vi "Loop_Auto.vi"() -> ()   [LabVIEW 2017, in "Autonomous.lvlib"]
uses:
  Autonomous.lvlib
  ENUM_Auto_State.ctl
  TypeDef/CLUSTER_CMD_WC_Drive.ctl
  TypeDef/ENUM_WC_Drive_DriveMode.ctl
  TypeDef/CLUSTER_Drive_ACT Loop_VBus Data.ctl
  TypeDef/CLUSTER_X and Y.ctl
  TypeDef/CLUSTER_Drive_ACT Loop_Profile Data.ctl
  ENUM_Auto_Action.ctl
  _SHARE ALL/Global Share All/Global_STOP.vi
  Globals/Global_CMD_Drive.vi
panel:
  out "Cycle Time (S)":dbl format="%.3g"
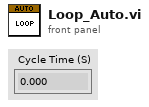
[diagram p1: front panel]
types:
  T1 = typedef "CLUSTER_CMD_WC_Drive.ctl" = cluster{"Drive_Mode":T2, "VBus":T3, "Profile":T5, "Zero Drive Encoders":bool, "Set Target Position(IN)":dbl, "Target Angle(Degree)":dbl, "Lock Angle":bool, "Zero YAW":bool}
  T2 = typedef "ENUM_WC_Drive_DriveMode.ctl" = enum16{"Motion Profile", "CrossLineAuto", "VBus", "Stop"}
  T3 = typedef "CLUSTER_Drive_ACT Loop_VBus Data.ctl" = cluster{"Drive":T4, "Turbo":bool}
  T4 = typedef "CLUSTER_X and Y.ctl" = cluster{"Steer":dbl, "Throtle":dbl}
  T5 = typedef "CLUSTER_Drive_ACT Loop_Profile Data.ctl" = cluster{"Start":bool}
  T6 = typedef "Autonomous.lvlib/ENUM_Auto_State.ctl" = enum16{"Startup", "Idle", "Cross Line", "Shutdown"}
  T7 = typedef "Autonomous.lvlib/ENUM_Auto_Action.ctl" = enum16{"No Action", "Reset Time", "Reset All", "Lock Angle", "Drive", "Zero Drive Encoders", "Zero YAW"}
  T8 = cluster{"State":T6, "Previous State":T6, "Current Time":timestamp, "Previous Time":timestamp, "Start Time":timestamp, "Target Time (ms)":u32, "Cycle Time(S)":dbl, "CMD_Drive_Data":T1, "Test":dbl, "Steering":dbl, "Throtal":dbl, "Encoder Target Position(in)":dbl, "Zero Drive Encoders":bool, "Lock Angle":bool, "Target Angle(Degree)":dbl, "Zero YAW":bool}
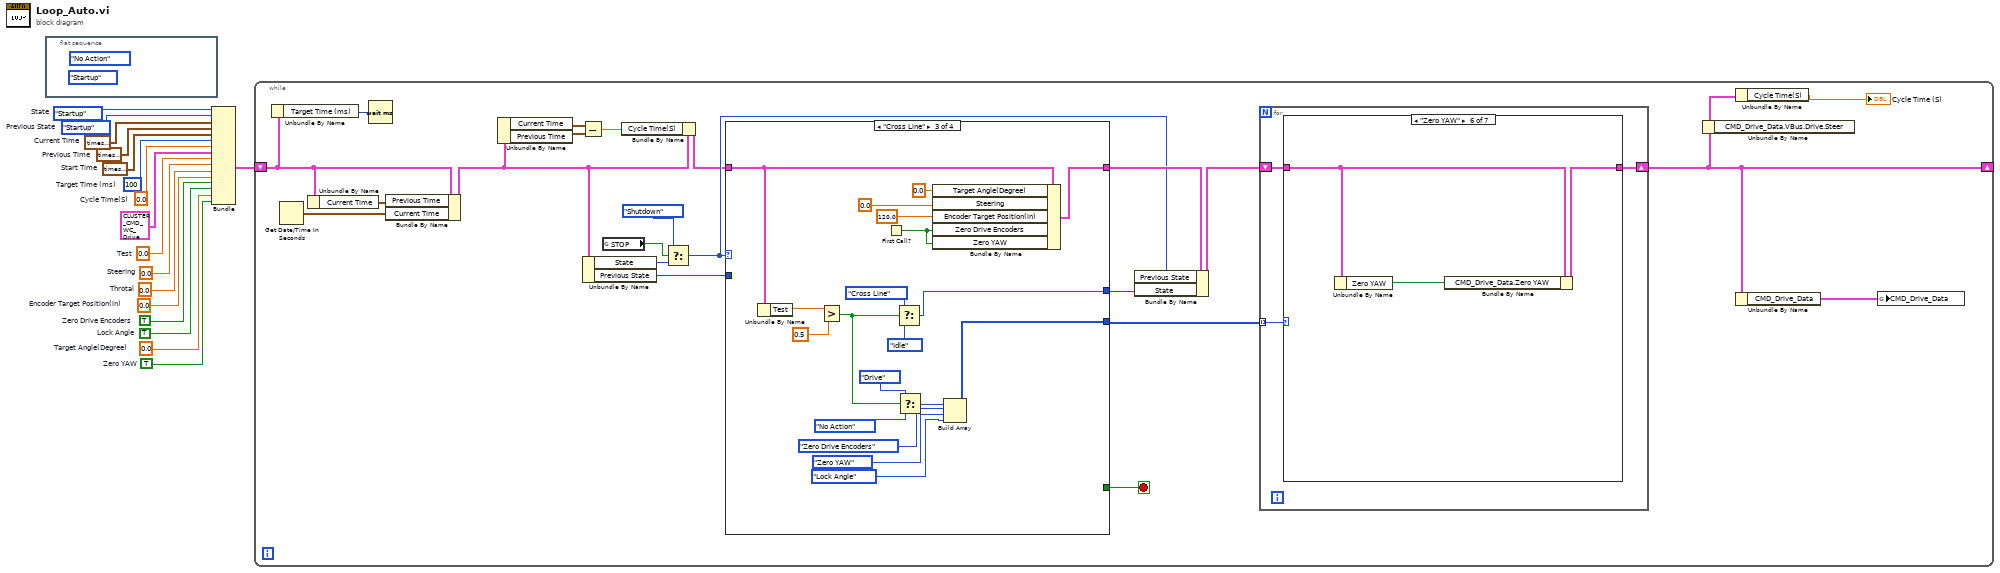
[diagram p0: block diagram]
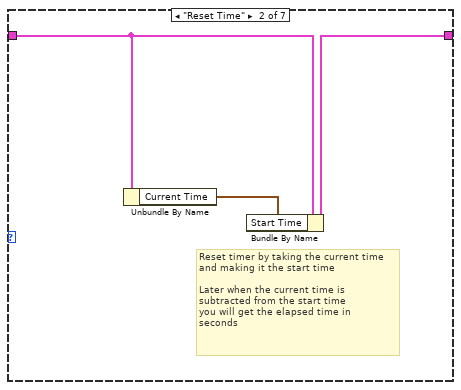
[diagram p3: hidden frame]
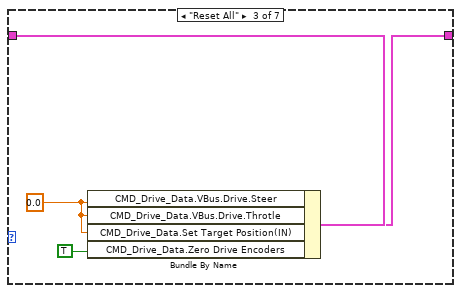
[diagram p4: hidden frame]
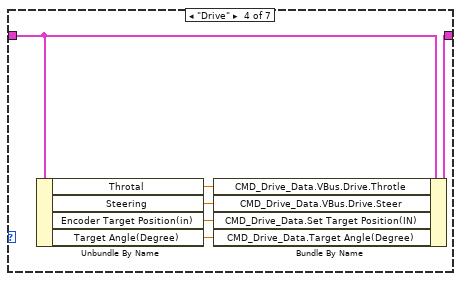
[diagram p5: hidden frame]
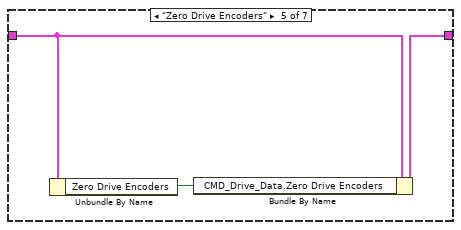
[diagram p6: hidden frame]
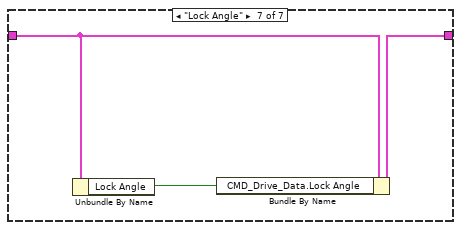
[diagram p7: hidden frame]
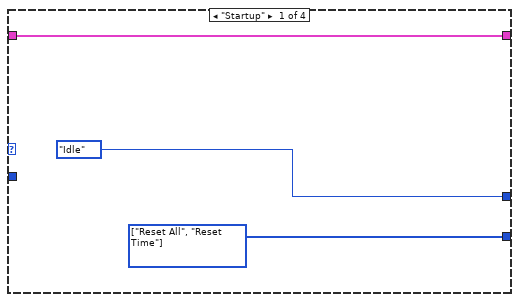
[diagram p8: hidden frame]
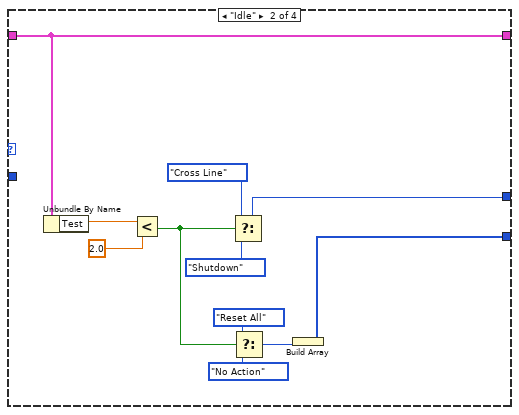
[diagram p9: hidden frame]
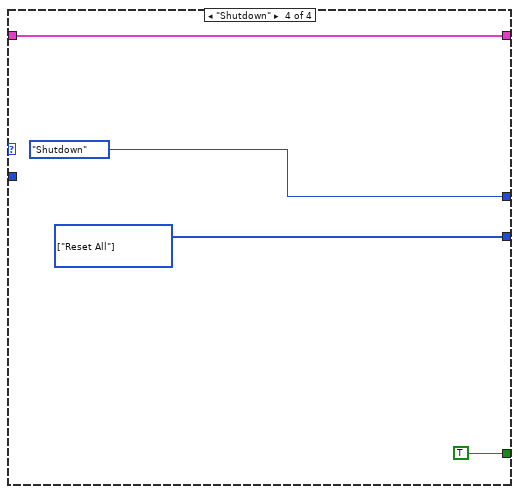
[diagram p10: hidden frame]
diagram:
  w1 = TRUE  # Zero YAW
  w2 = 0.0  # Target Angle(Degree)
  w3 = TRUE  # Lock Angle
  w4 = TRUE  # Zero Drive Encoders
  w5 = 0.0  # Encoder Target Position(in)
  w6 = 0.0  # Throtal
  w7 = 0.0  # Steering
  w8 = 0.0  # Test
  w10 = 0.0  # Cycle Time(S)
  w11 = ENUM_Auto_State."Startup"  # Previous State
  w12 = timestamp(0 s since 1904-01-01)  # Previous Time
  w13 = u32 100  # Target Time (ms)
  w14 = timestamp(0 s since 1904-01-01)  # Start Time
  w15 = timestamp(0 s since 1904-01-01)  # Current Time
  w16 = ENUM_Auto_State."Startup"  # State
  n1 = flat-sequence {
    frame #0 {
      (unwired) ENUM_Auto_State."Startup" ("State")
      (unwired) ENUM_Auto_Action."No Action" ("Action")
    }
  }
  n2 = Bundle("State"=w16, "Previous State"=w11, "Current Time"=w15, "Previous Time"=w12, "Start Time"=w14, "Target Time (ms)"=w13, "Cycle Time(S)"=w10, "CMD_Drive_Data"=T1 {"Drive_Mode"=enum."Motion Profile", "VBus"={"Drive"={"Steer"=0.0, "Throtle"=0.0}, "Turbo"=FALSE}, "Profile"={"Start"=FALSE}, "Zero Drive Encoders"=FALSE, "Set Target Position(IN)"=0.0, "Target Angle(Degree)"=0.0, "Lock Angle"=FALSE, "Zero YAW"=FALSE}, "Test"=w8, "Steering"=w7, "Throtal"=w6, "Encoder Target Position(in)"=w5, "Zero Drive Encoders"=w4, "Lock Angle"=w3, "Target Angle(Degree)"=w2, "Zero YAW"=w1) -> (w17:T8)  [unwired: 1 in]
  n3 = while {
    shift-right: [w27] -> _
    shift-left: w17 -> [w30]
    stop <- w19 stop-if-true
    n4 = Unbundle By Name(w30) -> ("Target Time (ms)"=w32:u32)
    n5 = Get Date/Time In Seconds() -> (seconds since 1Jan1904=w39:timestamp)
    n6 = Unbundle By Name(w30) -> ("Current Time"=w31:timestamp)
    n7 = Wait (ms)(milliseconds to wait=w32) -> ()  [unwired: 1 out]
    n8 = Bundle By Name(cluster=w30, "Previous Time"=w31, "Current Time"=w39) -> (w23:T8)
    n9 = Unbundle By Name(w23) -> ("Current Time"=w24:timestamp, "Previous Time"=w25:timestamp)
    n10 = Subtract(x=w24, y=w25) -> (x-y=w21:dbl)
    n11 = Unbundle By Name(w23) -> ("State"=w33:T6, "Previous State"=w29:T6)
    n12 = global read "Global_STOP.vi" "STOP"() -> (w35:bool)
    n13 = Bundle By Name(cluster=w23, "Cycle Time(S)"=w21) -> (w22:T8)
    n14 = Select(t=ENUM_Auto_State."Shutdown" ("State"), s=w35, f=w33) -> (s? t:f=w28:T6)
    n15 = case shown="\"Cross Line\"" w28 {
      tunnel: w22 -> [w68 w79 w88 w102]
      tunnel: [w68 w79 w87 w102] -> w37
      tunnel: [ENUM_Auto_State."Idle" ("State") w78 w98 ENUM_Auto_State."Shutdown" ("State")] -> w36
      tunnel: [w67 w71 w91 w100] -> w20
      tunnel: w29 -> [_ _ _ _]
      tunnel: [_ _ _ TRUE] -> w19
      frame "Startup" {
        w67 = T7[] [enum."Reset All", enum."Reset Time"] items=["No Action", "Reset Time", "Reset All", "Lock Angle", "Drive", "Zero Drive Encoders", "Zero YAW"] ("Actions")
      }
      frame "Idle" {
        n16 = Unbundle By Name(w79) -> ("Test"=w70:dbl)
        n17 = Less?(x=w70, y=2.0) -> (x < y?=w73:bool)
        n18 = Select(t=ENUM_Auto_State."Cross Line" ("State"), s=w73, f=ENUM_Auto_State."Shutdown" ("State")) -> (s? t:f=w78:T6)
        n19 = Select(t=ENUM_Auto_Action."Reset All" ("Action"), s=w73, f=ENUM_Auto_Action."No Action" ("Action")) -> (s? t:f=w72:T7)
        n20 = Build Array(w72) -> (w71:T7[])
      }
      frame "Cross Line" {
        n21 = Unbundle By Name(w88) -> ("Test"=w90:dbl)
        n22 = Greater?(x=w90, y=0.5) -> (0:w93:bool)
        n23 = First Call?() -> (First Call?: T/F=w82:bool)
        n24 = Select(t=ENUM_Auto_State."Cross Line" ("State"), s=w93, f=ENUM_Auto_State."Idle" ("State")) -> (s? t:f=w98:T6)
        n25 = Select(t=ENUM_Auto_Action."Drive" ("Action"), s=w93, f=ENUM_Auto_Action."No Action" ("Action")) -> (s? t:f=w92:T7)
        n26 = Bundle By Name(cluster=w88, "Target Angle(Degree)"=0.0, "Steering"=0.0, "Encoder Target Position(in)"=120.0, "Zero Drive Encoders"=w82, "Zero YAW"=w82) -> (w87:T8)
        n27 = Build Array(w92, ENUM_Auto_Action."Zero Drive Encoders" ("Action"), ENUM_Auto_Action."Zero YAW" ("Action"), ENUM_Auto_Action."Lock Angle" ("Action")) -> (w91:T7[])
      }
      frame "Shutdown" {
        w100 = T7[] [enum."Reset All"] items=["No Action", "Reset Time", "Reset All", "Lock Angle", "Drive", "Zero Drive Encoders", "Zero YAW"] ("Actions")
      }
    }
    n28 = Bundle By Name(cluster=w37, "Previous State"=w28, "State"=w36) -> (w38:T8)
    n29 = for {
      tunnel: w20 -> [w42] mode=indexing
      shift-right: [w41] -> w27
      shift-left: w38 -> [w40]
      n30 = case shown="\"Zero YAW\"" w42 {
        tunnel: w40 -> [w43 w46 w50 w56 w59 w62 w65]
        tunnel: [w43 w45 w49 w55 w58 w61 w64] -> w41
        frame "No Action" {
        }
        frame "Reset Time" {
          # "Reset timer by taking the current time\nand making it the start time\n\nLater when the current time is \nsubtracted from the start time\nyou will get the elapsed time in \nseconds"
          n31 = Unbundle By Name(w46) -> ("Current Time"=w44:timestamp)
          n32 = Bundle By Name(cluster=w46, "Start Time"=w44) -> (w45:T8)
        }
        frame "Reset All" {
          w48 = 0.0 ("FG Write Value")
          n33 = Bundle By Name(cluster=w50, "CMD_Drive_Data.VBus.Drive.Steer"=w48, "CMD_Drive_Data.VBus.Drive.Throtle"=w48, "CMD_Drive_Data.Set Target Position(IN)"=w48, "CMD_Drive_Data.Zero Drive Encoders"=TRUE ("Output Bool")) -> (w49:T8)
        }
        frame "Drive" {
          n34 = Unbundle By Name(w56) -> ("Throtal"=w54:dbl, "Steering"=w53:dbl, "Encoder Target Position(in)"=w52:dbl, "Target Angle(Degree)"=w51:dbl)
          n35 = Bundle By Name(cluster=w56, "CMD_Drive_Data.VBus.Drive.Throtle"=w54, "CMD_Drive_Data.VBus.Drive.Steer"=w53, "CMD_Drive_Data.Set Target Position(IN)"=w52, "CMD_Drive_Data.Target Angle(Degree)"=w51) -> (w55:T8)
        }
        frame "Zero Drive Encoders" {
          n36 = Unbundle By Name(w59) -> ("Zero Drive Encoders"=w57:bool)
          n37 = Bundle By Name(cluster=w59, "CMD_Drive_Data.Zero Drive Encoders"=w57) -> (w58:T8)
        }
        frame "Zero YAW" {
          n38 = Unbundle By Name(w62) -> ("Zero YAW"=w60:bool)
          n39 = Bundle By Name(cluster=w62, "CMD_Drive_Data.Zero YAW"=w60) -> (w61:T8)
        }
        frame "Lock Angle" {
          n40 = Unbundle By Name(w65) -> ("Lock Angle"=w63:bool)
          n41 = Bundle By Name(cluster=w65, "CMD_Drive_Data.Lock Angle"=w63) -> (w64:T8)
        }
      }
    }
    n42 = Unbundle By Name(w27) -> ()  [unwired: 1 out]
    n43 = Unbundle By Name(w27) -> ("Cycle Time(S)"=→"Cycle Time (S)":dbl)
    n44 = Unbundle By Name(w27) -> ("CMD_Drive_Data"=w18:T1)
    n45 = global write "Global_CMD_Drive.vi" "CMD_Drive_Data"(w18) -> ()
  }
